vi "Reports_ParseArray.vi"(8 "error in (no error)":errorcluster, 9 "Array Req#":string[](array[string])=["309", "365", "279", "308", "468", "506", "385", "269", "396", "276", "364", "330", "273", "465", "474", "301", "335"], 11 "Array Req & Notes":string[][](array[string])=[["309", "Reset ip, safe mode and no app, where able to find the cRIO and format. That should take care of the slow deployment. "], ["365", "Needed to change the battery. "], ["279", "No Wireless allowed"], ["308", "Found material"], ["269", "Didnt need help. "], ["396", "Version 47"], ["276", "Reformatted controller and now deployment time is as expected."], ["364", "Axis camera was not on same subnet as computer. Once it was set to the correct IP address with the camera tool, they were able to see the image in the driver station. "], ["330", "Needed help with timing for autonomous mode. Told them about timing vis and flat sequence structures. "], ["273", "ni.com/frc for labview examples and training. also help in labview toolbar and then find examples "], ["301", "Changed sidecar"], ["335", "Done"]]) -> (0 "error out":errorcluster, 3 "Spaced Array":string[](array[string]))   [LabVIEW 2014, in "FIRST Reports.lvlib"]
uses:
  FIRST Reports.lvlib
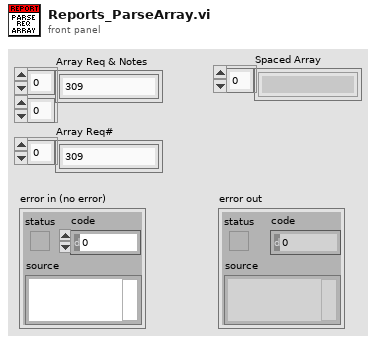
[diagram p1: front panel]
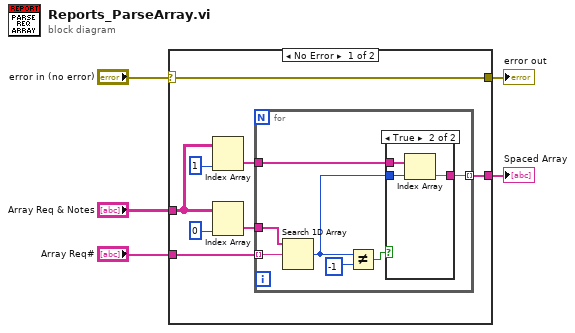
[diagram p0: block diagram]
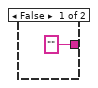
[diagram p2: hidden frame]
diagram:
  n1 = case shown="No Error" "error in (no error)" {
    selector: "error in (no error)" -> [w6 w25]
    tunnel: [w6 w25] -> w5
    tunnel: "Array Req & Notes" -> [w9 _]
    tunnel: "Array Req#" -> [w8 _]
    tunnel: [w7 _] -> w1
    frame No Error {
      n2 = Index Array(array=w9, index (col)=1 ("disabled index (col)")) -> (element=w13:string[])  [unwired: 1 in]
      n3 = Index Array(array=w9, index (col)=0 ("disabled index (col)")) -> (element=w12:string[])  [unwired: 1 in]
      n4 = for {
        tunnel: w8 -> [w19] mode=indexing
        tunnel: w12 -> [w20]
        tunnel: w13 -> [w15]
        tunnel: [w14] -> w7 mode=indexing
        n5 = Search 1D Array(1D array=w20, element=w19) -> (index of element=w16:i32)  [unwired: 1 in]
        n6 = Not Equal?(x=w16, y=-1) -> (x != y?=w17:bool)
        n7 = case shown="True" w17 {
          tunnel: w16 -> [_ w23]
          tunnel: w15 -> [_ w24]
          tunnel: ["" ("format string") w22] -> w14
          frame False {
          }
          frame True {
            n8 = Index Array(array=w24, index=w23) -> (element=w22:string)
          }
        }
      }
    }
    frame Error {
    }
  }
  "error out" <- w5
  "Spaced Array" <- w1
